vi "Get Data Log File Settings.vi"(8 "error in":errorcluster, 11 "File Ref in":T1 format="%.0x") -> (0 "error out":errorcluster, 1 "Pretrigger Samples":i32, 2 "File Log Specification":T2={"Directory"=path "", "Groups"=[], "Buffer Size"=0, "Properties"=[], "Pretrigger"=FALSE, "Pretrigger Samples"=0, "Name"="", "Timestamp"=FALSE, "Error"=0, "Auto Open"=FALSE, "File Node Ref"=18446744073709551615, "Archive"=FALSE, "Archive Directory"=path "", "Segment Files"=FALSE, "Segment Files By"=enum."Size", "Segment Size"=100000, "Flushed Data Size Total"=0, "Append Waveform Properties"=FALSE, "Logging State"=enum."Not Started", "First Sample Start Time"=timestamp(0 s since 1904-01-01), "System dt"=0.0} {"File Node Ref" format="%.0x"}, 3 "File Ref Out":T1 format="%.0x", 4 "System dt":dbl)   [LabVIEW 2027, in "Embedded Data Logger Engine.lvlib"]
uses:
  Embedded Data Logger Engine.lvlib
  <vilib>/NI VeriStand/Custom Device API/Custom Device Item Ref.ctl
  File Logging Specification.ctl
  Group Logging Specification.ctl
  Group Buffer Data.ctl
  Property Specification.ctl
  Shared/Segment Files By.ctl
  Logging State.ctl
  <vilib>/NI VeriStand/Custom Device API/Custom Device API.lvlib
  Scripting/Embedded Data Logger Scripting.lvlib
  Shared/Embedded Data Logger Shared.lvlib
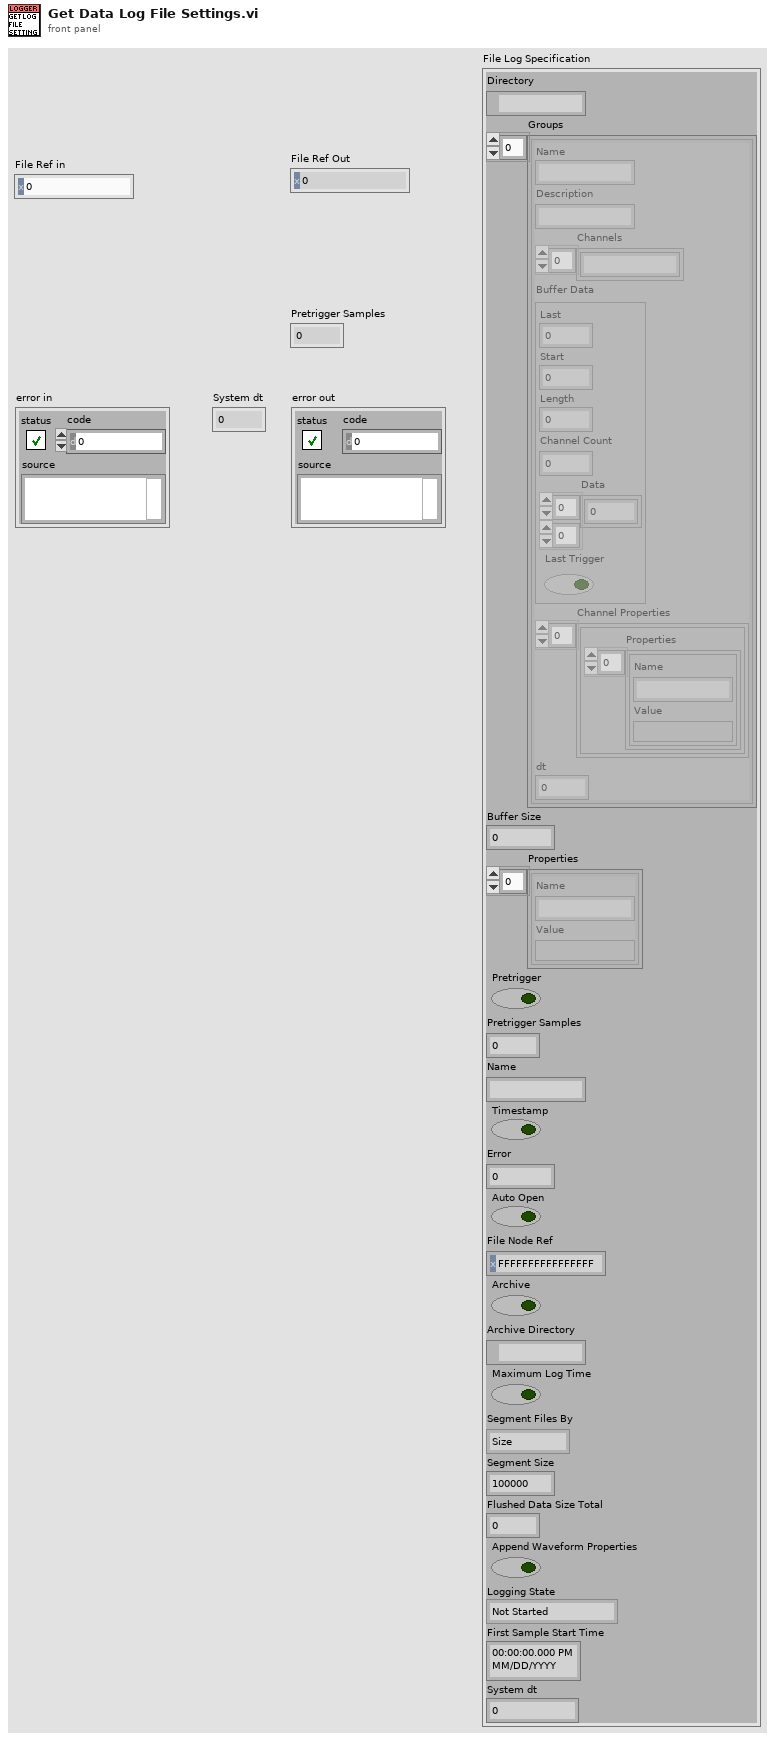
[diagram p1: front panel]
types:
  T1 = typedef "Custom Device API.lvlib/Custom Device Item Ref.ctl" = u64
  T2 = typedef "Embedded Data Logger Engine.lvlib/File Logging Specification.ctl" = cluster{"Directory":path, "Groups":T3[], "Buffer Size":i32, "Properties":T5[], "Pretrigger":bool, "Pretrigger Samples":i32, "Name":string, "Timestamp":bool, "Error":i32, "Auto Open":bool, "File Node Ref":T1, "Archive":bool, "Archive Directory":path, "Segment Files":bool, "Segment Files By":T6, "Segment Size":u32, "Flushed Data Size Total":u32, "Append Waveform Properties":bool, "Logging State":T7, "First Sample Start Time":timestamp, "System dt":dbl}
  T3 = typedef "Embedded Data Logger Engine.lvlib/Group Logging Specification.ctl" = cluster{"Name":string, "Description":string, "Channels":string[], "Buffer Data":T4, "Channel Properties":cluster{"Properties":T5[]}[], "dt":dbl}
  T4 = typedef "Embedded Data Logger Engine.lvlib/Group Buffer Data.ctl" = cluster{"Last":i32, "Start":i32, "Length":i32, "Channel Count":i32, "Data":dbl[][], "Last Trigger":bool}
  T5 = typedef "Embedded Data Logger Engine.lvlib/Property Specification.ctl" = cluster{"Name":string, "Value":variant}
  T6 = typedef "Embedded Data Logger Shared.lvlib/Segment Files By.ctl" = enum16{"Time", "Size"}
  T7 = typedef "Embedded Data Logger Engine.lvlib/Logging State.ctl" = enum16{"Not Started", "Continous Logging", "Paused", "Discontinous Logging"}
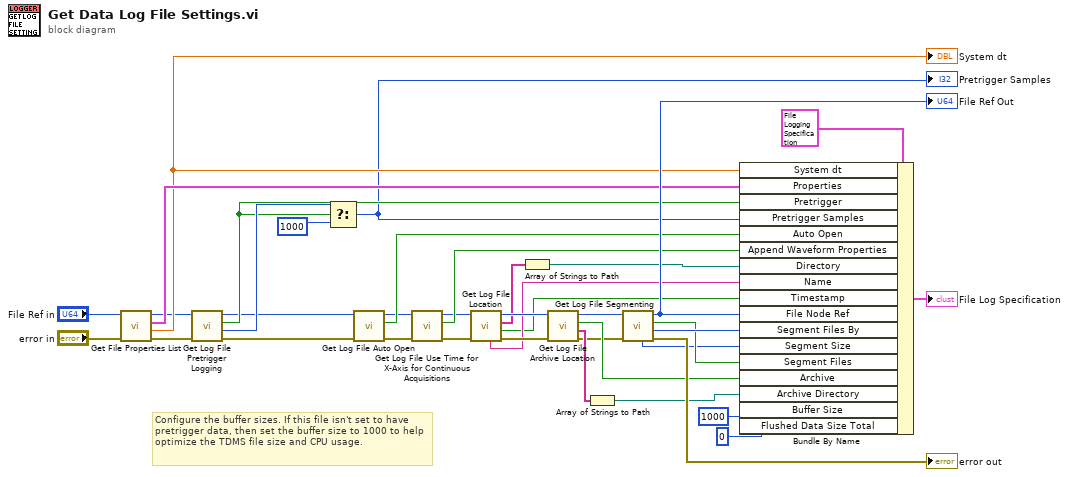
[diagram p0: block diagram]
diagram:
  # "Configure the buffer sizes. If this file isn't set to have pretrigger data, then set the buffer size to 1000 to help optimize the TDMS file size and CPU usage."
  n1 = call "Get File Properties List.vi"("error in (no error)"="error in", "File Ref in"="File Ref in") -> ("error out"=w25:errorcluster, "System dt"=w29:dbl, "Properties List"=w33:T5[], "File Ref out"=w20:T1)  [unwired: 6 out]
  "System dt" <- w29
  n2 = call "Get Log File Pretrigger Logging.vi"("error in"=w25, "log file in"=w20) -> ("error out"=w18:errorcluster, "pretrigger samples"=w24:i32, "pretrigger logging"=w22:bool, "log file out"=w19:T1)  [unwired: 6 in]
  n3 = Select(t=w24, s=w22, f=1000) -> (s? t:f=w21:i32)
  "Pretrigger Samples" <- w21
  n4 = call "Get Log File Auto Open.vi"("error in"=w18, "log file in"=w19) -> ("error out"=w15:errorcluster, "auto open"=w17:bool, "log file out"=w16:T1)  [unwired: 7 in]
  n5 = call "Get Log File Use Time for X-Axis for Continuous Acquisitions.vi"("error in"=w15, "log file in"=w16) -> ("error out"=w10:errorcluster, "use time for x-axis for continuous acquisitions"=w14:bool, "log file out"=w11:T1)  [unwired: 7 in]
  n6 = call "Get Log File Location.vi"("error in (no error)"=w10, "log file in"=w11) -> ("error out"=w13:errorcluster, "timestamp file name"=w6:bool, "directory parts"=w8:string[], "log file out"=w12:T1, "base file name"=w7:string)  [unwired: 4 in, 1 out]
  n7 = Array of Strings to Path(0:w8) -> (2:w9:path)  [unwired: 1 in]
  n8 = call "Get Log File Archive Location.vi"("error in (no error)"=w13, "log file in"=w12) -> ("error out"=w1:errorcluster, "archive directory parts"=w5:string[], "archive closed log files"=w3:bool, "log file out"=w2:T1)  [unwired: 6 in]
  n9 = Array of Strings to Path(0:w5) -> (2:w4:path)  [unwired: 1 in]
  n10 = call "Get Log File Segmenting.vi"("error in"=w1, "log file in"=w2) -> ("error out"=→"error out":errorcluster, "file segmenting mode"=w28:T6, "segment into multiple files"=w27:bool, "log file out"=w36:T1, "file length (s) or size (MB)"=w26:u32)  [unwired: 5 in]
  "File Ref Out" <- w36
  n11 = Bundle By Name(cluster=T2 {"Directory"=path "", "Groups"=[], "Buffer Size"=0, "Properties"=[], "Pretrigger"=FALSE, "Pretrigger Samples"=0, "Name"="", "Timestamp"=FALSE, "Error"=0, "Auto Open"=FALSE, "File Node Ref"=18446744073709551615, "Archive"=FALSE, "Archive Directory"=path "", "Segment Files"=FALSE, "Segment Files By"=enum."Time", "Segment Size"=0, "Flushed Data Size Total"=0, "Append Waveform Properties"=FALSE, "Logging State"=enum."Not Started", "First Sample Start Time"=timestamp(0 s since 1904-01-01), "System dt"=0.0} ("File Log Spec"), "System dt"=w29, "Properties"=w33, "Pretrigger"=w22, "Pretrigger Samples"=w21, "Auto Open"=w17, "Append Waveform Properties"=w14, "Directory"=w9, "Name"=w7, "Timestamp"=w6, "File Node Ref"=w36, "Segment Files By"=w28, "Segment Size"=w26, "Segment Files"=w27, "Archive"=w3, "Archive Directory"=w4, "Buffer Size"=1000, "Flushed Data Size Total"=u32 0) -> (→"File Log Specification":T2)
